vi "Analysis.Result Summaries, TE, Gen Paredo Table.vi"(11 "Test History":T3) -> ()   [LabVIEW 2024]
uses:
  TestExec/TestExec.Test Result Metric History.ctl
  TestExec/TestExec.Test Result Metric History Item.ctl
  <vilib>/KATE/SeqMgr/SeqMgr.Result State Enum.ctl
  Analysis.Result Summary, Metrics.ctl
  Analysis.Result Summary.ctl
  <vilib>/KATE/SeqMgr/SeqMgr.lvlib
panel:
  out "Test Time Histogram":T1(graph)
  out "Test Times (s)":cluster{"Min":dbl, "Max":dbl, "Avg":dbl}
  out "Metrics":T2 {"Yield%" format="%.2f"}
  out "FP Pareto":string[][](table)
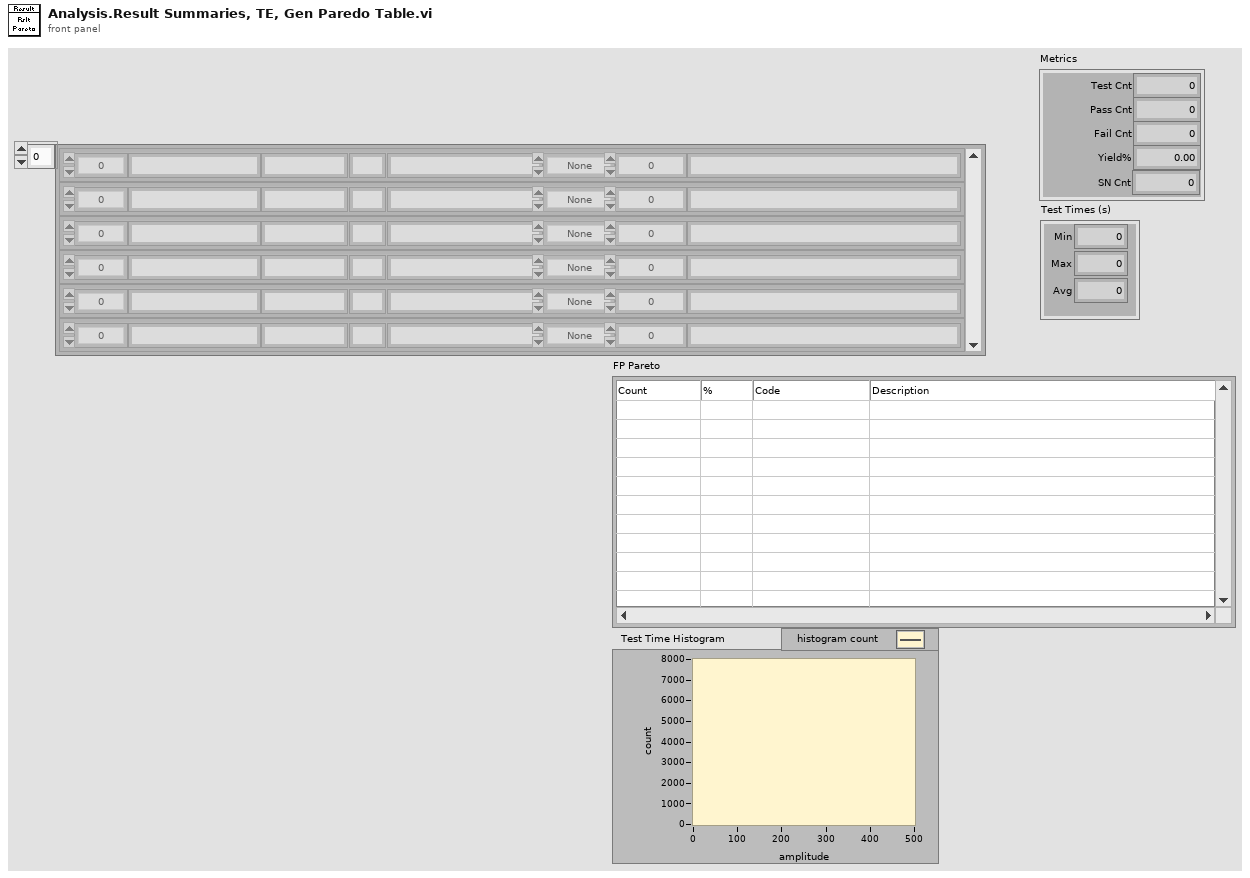
[diagram p1: front panel]
types:
  T1 = cluster{"X Values":dbl[], "Histogram: h(x)":i32[]}
  T2 = typedef "Analysis.Result Summary, Metrics.ctl" = cluster{"Pass Cnt":i32, "Fail Cnt":i32, "Yield%":dbl, "Test Cnt":i32, "SN Cnt":i32}
  T3 = typedef "TestExec.Test Result Metric History.ctl" = T4[]
  T4 = typedef "TestExec.Test Result Metric History Item.ctl" = cluster{"TimeStamp":timestamp, "Dur(s)":dbl, "Time":string, "Mode ":string, "Test ":string, "SN":string, "State":T5, "Code":i32, "Description":string, "Pos ":string}
  T5 = typedef "KATE_Lib.lvlib/SeqMgr.lvlib/SeqMgr.Result State Enum.ctl" = enum16{"None", "Passing", "Failing", "PASS", "FAIL", "ABORT", "ERROR"}
  T6 = typedef "Analysis.Result Summary.ctl" = cluster{"SN":string, "Start Time":timestamp, "Location":string, "Nest":string, "Sequence":string, "Operator":string, "Test Mode":string, "Comment":string, "Result":string, "Result Code":i32, "Result Desc":string, "Date":string, "Dur(s)":dbl, "PASS":bool, "FirstPass":bool, "LastPass":bool, "LocationID":i32, "ModeID":i32, "SeqID":i32, "RsltID":i32, "Genealogy":string[][]}
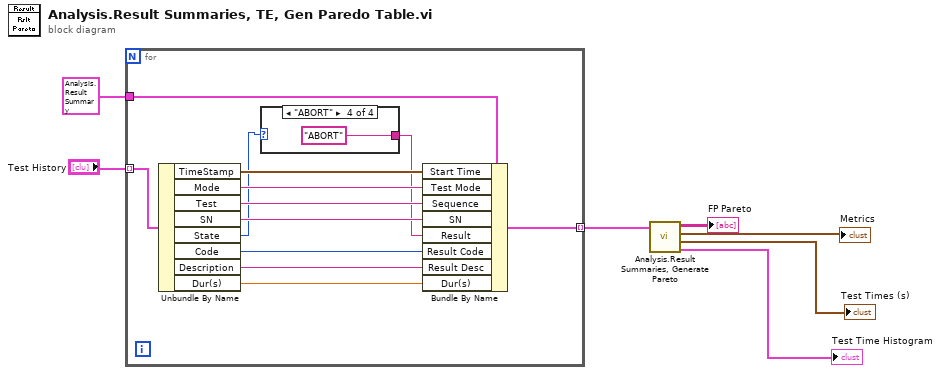
[diagram p0: block diagram]
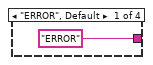
[diagram p2: hidden frame]
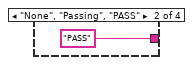
[diagram p3: hidden frame]
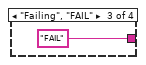
[diagram p4: hidden frame]
diagram:
  n1 = for {
    tunnel: "Test History" -> [w19] mode=indexing
    tunnel: T6 {"SN"="", "Start Time"=timestamp(0 s since 1904-01-01), "Location"="", "Nest"="", "Sequence"="", "Operator"="", "Test Mode"="", "Comment"="", "Result"="", "Result Code"=0, "Result Desc"="", "Date"="", "Dur(s)"=0.0, "PASS"=FALSE, "FirstPass"=FALSE, "LastPass"=FALSE, "LocationID"=0, "ModeID"=0, "SeqID"=0, "RsltID"=0, "Genealogy"=[]} ("Result Summary") -> [w18]
    tunnel: [w8] -> w5 mode=indexing
    n2 = Unbundle By Name(w19) -> ("TimeStamp"=w17:timestamp, "Mode"=w16:string, "Test"=w15:string, "SN"=w14:string, "State"=w12:T5, "Code"=w13:i32, "Description"=w10:string, "Dur(s)"=w9:dbl)
    n3 = case shown="\"ABORT\"" w12 {
      tunnel: ["ERROR" "PASS" "FAIL" "ABORT"] -> w11
      frame "ERROR", Default {
      }
      frame "None", "Passing", "PASS" {
      }
      frame "Failing", "FAIL" {
      }
      frame "ABORT" {
      }
    }
    n4 = Bundle By Name(cluster=w18, "Start Time"=w17, "Test Mode"=w16, "Sequence"=w15, "SN"=w14, "Result"=w11, "Result Code"=w13, "Result Desc"=w10, "Dur(s)"=w9) -> (w8:T6)
  }
  n5 = call "Analysis.Result Summaries, Generate Pareto.vi"("ResultSum"=w5) -> ("Test Time Histogram"=→"Test Time Histogram":T1, "Test Times (s)"=→"Test Times (s)":cluster{"Min":dbl, "Max":dbl, "Avg":dbl}, "Metrics"=→"Metrics":T2, "FP Pareto"=→"FP Pareto":string[][])  [unwired: 7 in]
